vi "Select Result File Path from ResultsDB.vi"(8 "error in (no error)":errorcluster, 10 "StationName":string, 11 "Barcode":string) -> (0 "error out":errorcluster, 2 "StationName List":string[](array[string]), 3 "Path":path)   [LabVIEW 2021, in "SQLite.lvclass"]
doc: "Get waveform file path depend on station name and Barcode."
uses:
  SQLite.lvclass
  SQLite.lvclass/SQLite.ctl
  <userlib>/LabSQL/LabSQL.lvlib
  vi.lib_New/TopPath/TopPath.lvlib
panel:
  out "Table Control":string[][](table)
  out "Select SQL CMD":string
  out "number (0 to 1)":dbl
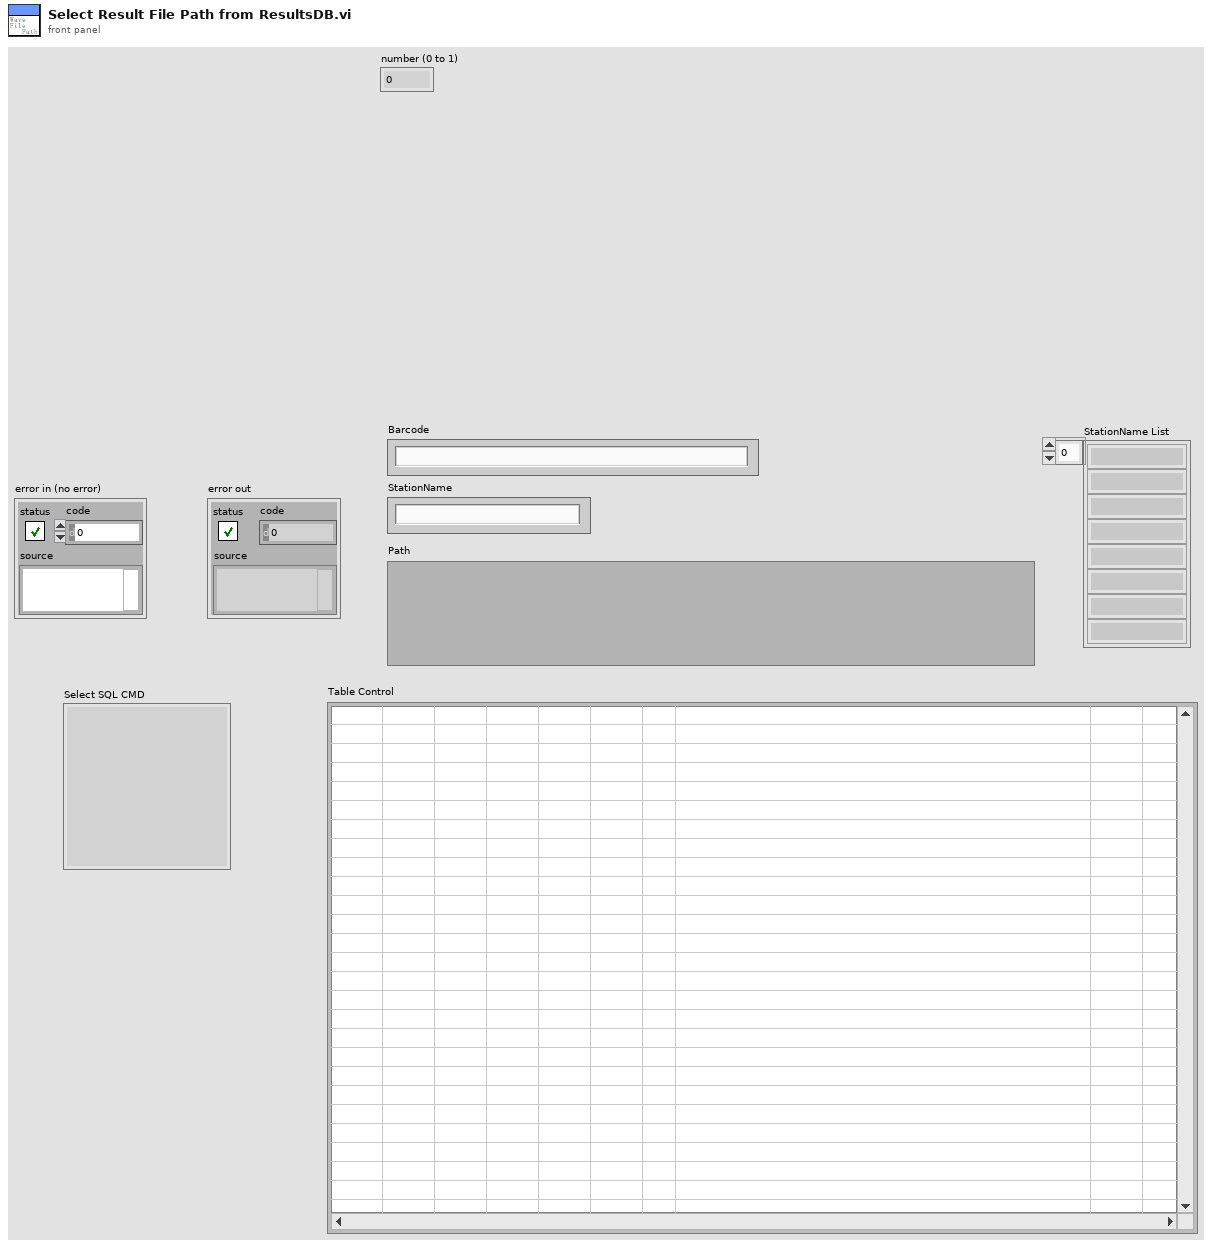
[diagram p1: front panel]
types:
  T1 = enum16{"Other", "SQL2008", "SQLite", "Access", "MySQL"}
  T2 = typedef "TopPath.lvlib/Top Path.ctl" = cluster{"LV Source":path, "FilePath":path, "Data":path}
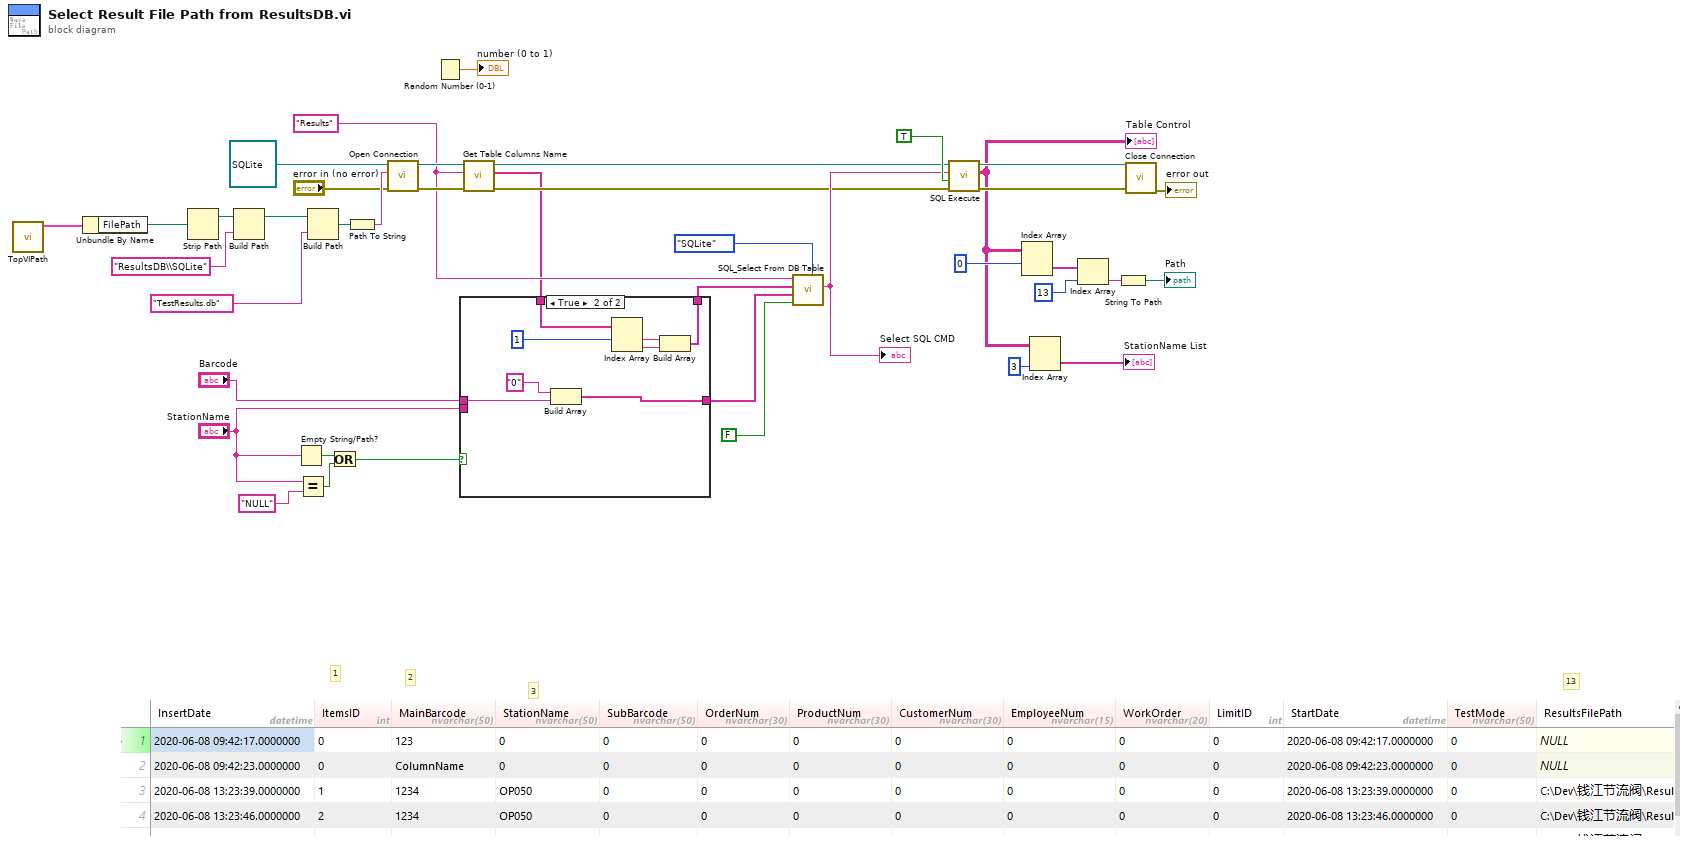
[diagram p0: block diagram]
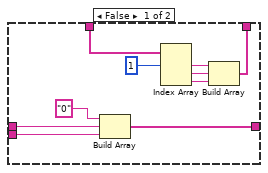
[diagram p2: hidden frame]
diagram:
  w21 = "Results" ("TableName")
  # "1"
  # "13"
  # "3"
  # "2"
  n1 = call "TopVIPath.vi"() -> ("TopPath"=w39:T2)  [unwired: 10 in, 1 out]
  n2 = Unbundle By Name(w39) -> ("FilePath"=w38:path)
  n3 = Strip Path(path=w38) -> (stripped path=w37:path)  [unwired: 1 out]
  n4 = Build Path(base path=w37, name or relative path="ResultsDB\\SQLite") -> (appended path=w35:path)
  n5 = Empty String/Path?(string/path="StationName") -> (empty?=w6:bool)
  n6 = Equal?(x="StationName", y="NULL") -> (x = y?=w5:bool)
  n7 = Build Path(base path=w35, name or relative path="TestResults.db") -> (appended path=w30:path)
  n8 = Or(x=w6, y=w5) -> (x .or. y?=w4:bool)
  n9 = Path To String(path=w30) -> (string=w29:string)
  n10 = call-dynamic "Open Connection.vi"("error in (no error)"="error in (no error)", "ConnectionString"=w29, "HostDB in"=refnum<class "SQLite.lvclass"> refnum ("SQLite.lvclass")) -> ("error out"=w33:errorcluster, "HostDB out"=w32:refnum<class "SQLite.lvclass">)  [unwired: 7 in]
  n11 = Random Number (0-1)() -> (number: 0 to 1=→"number (0 to 1)":dbl)
  n12 = call-dynamic "Get Table Columns Name.vi"("error in (no error)"=w33, "TableName"=w21, "HostDB in"=w32) -> ("error out"=w18:errorcluster, "Table_ColunmsList"=w16:string[], "HostDB out"=w20:refnum<class "SQLite.lvclass">)  [unwired: 4 in, 2 out]
  n13 = case shown="True" w4 {
    tunnel: [w50 w58] -> w22
    tunnel: w16 -> [w49 w57]
    tunnel: [w45 w53] -> w15
    tunnel: "Barcode" -> [w44 w52]
    tunnel: "StationName" -> [w41 _]
    frame False {
      n14 = Build Array("0" ("element"), w44, w41) -> (w50:string[])
      n15 = Index Array(array=w49, index #1=1 ("index")) -> (element #1=w47:string, element #2=w46:string, element #3=w43:string)  [unwired: 2 in]
      n16 = Build Array(w47, w46, w43) -> (w45:string[])
    }
    frame True {
      n17 = Build Array("0" ("element"), w52) -> (w58:string[])
      n18 = Index Array(array=w57, index #1=1 ("index")) -> (element #1=w55:string, element #2=w54:string)  [unwired: 1 in]
      n19 = Build Array(w55, w54) -> (w53:string[])
    }
  }
  n20 = call <userlib>:"SQL_Select From DB Table.vi"("DB Type"=T1."SQLite", "Check ASCII?"=FALSE, "ColumnsValue"=w22, "ColumnsNameList"=w15, "TableName"=w21) -> ("Select SQL CMD"=w24:string)  [unwired: 6 in]
  "Select SQL CMD" <- w24
  n21 = call-dynamic "SQL Execute.vi"("error in (no error)"=w18, "Return Data (T)"=TRUE, "Command Text"=w24, "HostDB in"=w20) -> ("error out"=w17:errorcluster, "Table Control"=w3:string[][], "HostDB out"=w19:refnum<class "SQLite.lvclass">)  [unwired: 3 in, 2 out]
  "Table Control" <- w3
  n22 = Index Array(array=w3, index (row)=0) -> (element=w12:string[])  [unwired: 1 in]
  n23 = Index Array(array=w3, index (col)=3 ("disabled index (col)")) -> (element=→"StationName List":string[])  [unwired: 1 in]
  n24 = Index Array(array=w12, index=13) -> (element=w10:string)
  n25 = String To Path(string=w10) -> (path=→"Path":path)
  n26 = call-dynamic "Close Connection.vi"("error in (no error)"=w17, "HostDB in"=w19) -> ("error out"=→"error out":errorcluster)  [unwired: 8 in, 1 out]
